vi "Convert_UI_ERD_RT.vi"(0 "New Header?":bool, 2 "ERD Name":string[](array[string]), 5 "All_Bundled_Data_Brass":T1, 7 "Array":T8[](array[typedef]) {"ERD Number" format="%.0x"}, 11 "Error In":errorcluster) -> (6 "All_ERD_Data_Bundled_Brass":T1, 15 "Error Out":errorcluster)   [LabVIEW 2021]
doc: "This VI parses the data from ERDs in correct format, units, etc. It handles all hex to dec conversions, hex to enum, and hex to boolean conversions.\n\nIf Raw Data from ERD is blank string, then it will output values from shift register."
uses:
  Common/LabVIEW GEA2 Toolkit/GEA3/type defs/ERD Read Data Out.ctl
  Controls/All_Bundled_Data_RT.ctl
  Dryer Tool (Commercial 2)/JL Dryer Tool Support/type defs/Version.ctl
  Dryer Tool (Commercial 2)/JL Dryer Tool Support/type defs/ERD_Always_Show_JL.ctl
  Dryer Tool (Commercial 2)/JL Dryer Tool Support/type defs/CSV_File_String_Arrays.ctl
  Dryer Tool (Commercial 2)/JL Dryer Tool Support/type defs/Fault Table Array.ctl
  Dryer Tool (Commercial 2)/JL Dryer Tool Support/type defs/Fault_Table_Info.ctl
  Dryer Tool (Commercial 2)/JL Dryer Tool Support/type defs/BootloaderVersion.ctl
panel:
  out "ERD Number":u16 format="%x"
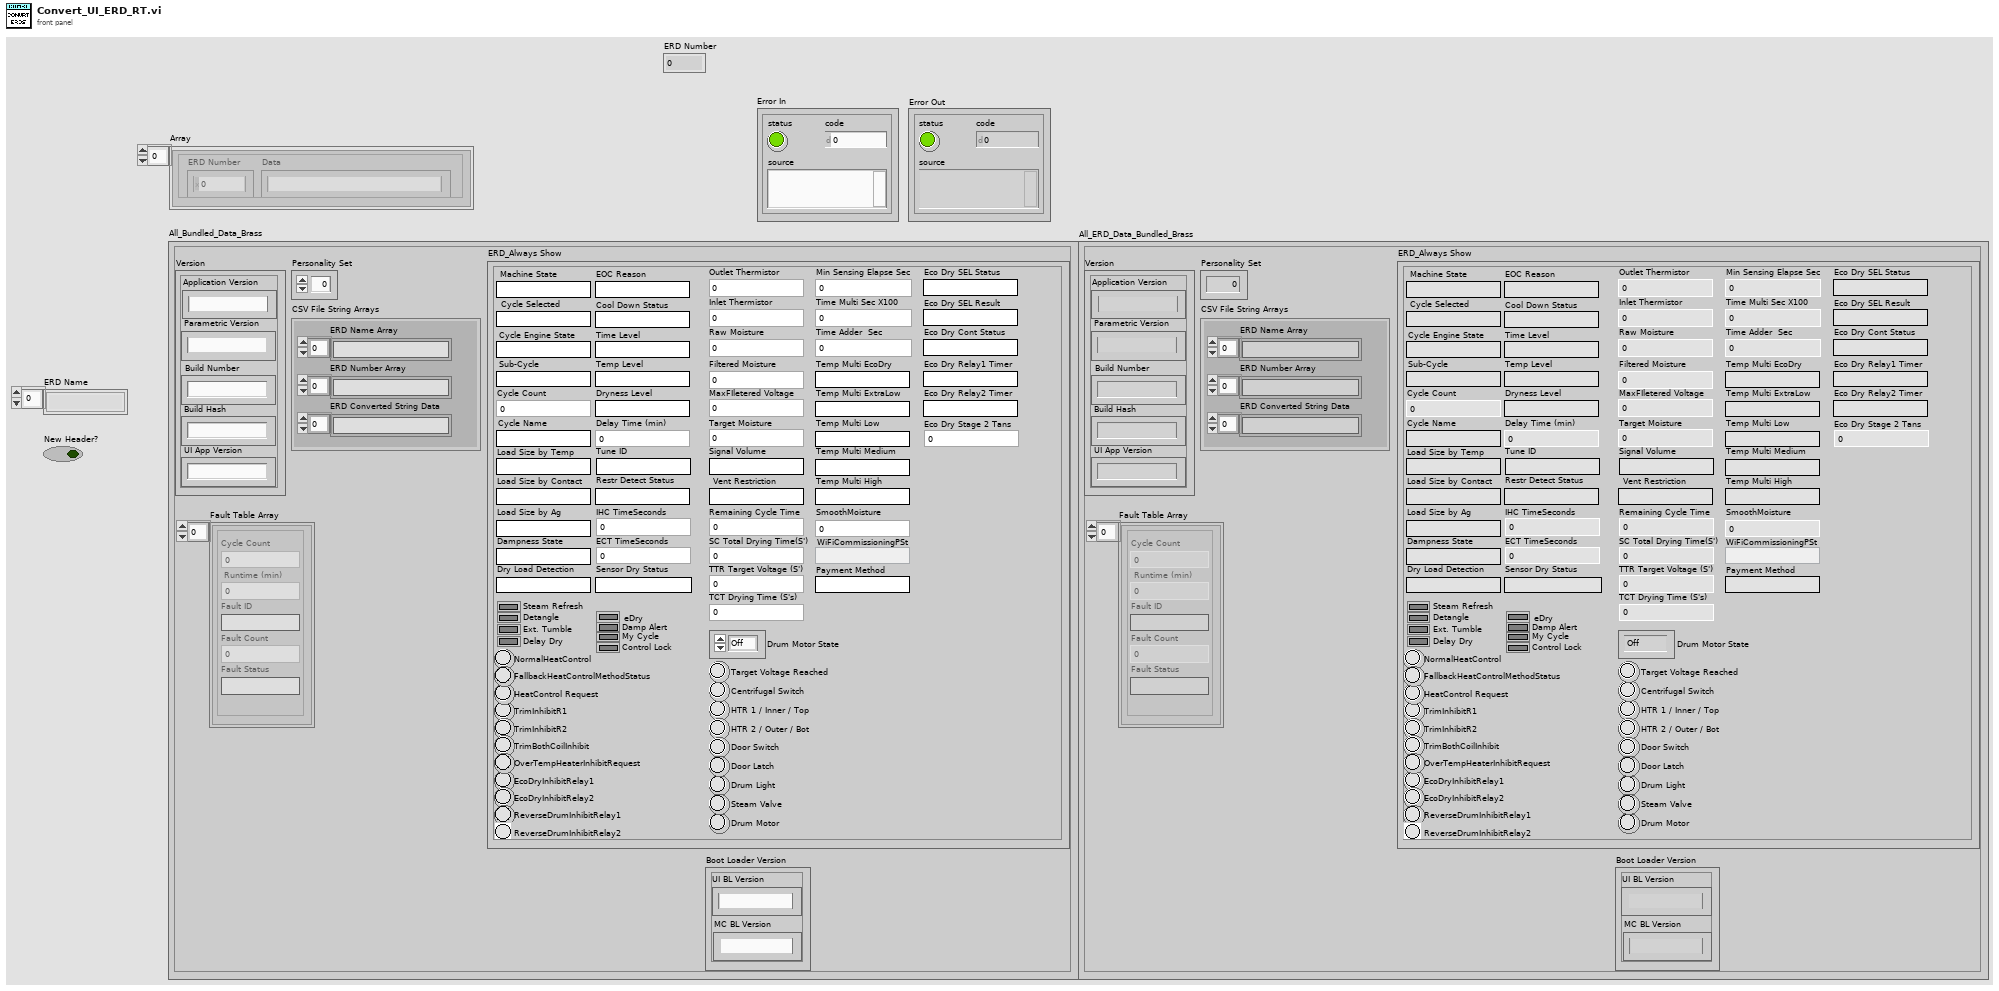
[diagram p1: front panel]
types:
  T1 = typedef "All_Bundled_Data_RT.ctl" = cluster{"Version":T2, "ERD_Always Show":T3, "Personality Set":u8, "CSV File String Arrays":T4, "Fault Table Array ":T5, "Boot Loader Version":T7}
  T2 = typedef "Version.ctl" = cluster{"Build Number":string, "Build Hash ":string, "Application Version":string, "Parametric Version":string, "UI App Version":string}
  T3 = typedef "ERD_Always_Show_JL.ctl" = cluster{"Inlet Thermistor":u16, "Machine State":string, "Filtered Moisture":u16, "Cycle Selected":string, "HTR 1 / Inner / Top":bool, "HTR 2 / Outer / Bot":bool, "Door Switch":bool, "Drum Light":bool, "Cycle Engine State":string, "Centrifugal Switch":bool, "Drum Motor":bool, "Cycle Count":u32, "Ext. Tumble":bool, "eDry":bool, "Temp Level":string, "Dryness Level":string, "Time Level":string, "Delay Time (min)":u16, "Steam Refresh":bool, "Damp Alert":bool, "Sub-Cycle":string, "Outlet Thermistor":u16, "Target Moisture":u16, "Remaining Cycle Time":u32, "Raw Moisture":u16, "Cycle Name":string, "My Cycle":bool, "Delay Dry":bool, "Detangle":bool, "Control Lock":bool, "Steam Valve":bool, "Door Latch":bool, "Signal Volume":string, "Tune ID":string, "Restr Detect Status":string, "Vent Restriction":string, "Load Size by Contact":string, "Load Size by Temp":string, "EOC Reason":string, "Sensor Dry Status":string, "Dampness State":string, "Target Voltage Reached":bool, "TrimInhibitR1":bool, "TrimInhibitR2":bool, "TrimBothCoilInhibit":bool, "NormalHeatControl":bool, "HeatControl Request":bool, "Cool Down Status":string, "EcoDryInhibitRelay1":bool, "EcoDryInhibitRelay2":bool, "ReverseDrumInhibitRelay1":bool, "ReverseDrumInhibitRelay2":bool, "OverTempHeaterInhibitRequest":bool, "FallbackHeatControlMethodStatus":bool, "IHC TimeSeconds":u32, "ECT TimeSeconds ":u32, "SC Total Drying Time(S')":u32, "TTR Target Voltage (S')":u32, "TCT Drying Time (S's)":u32, "Drum Motor State":enum16{"Off", "Cw", "Ccw", "Max"}, "Load Size by Ag":string, "MaxFIletered Voltage":u16, "Dry Load Detection":string, "Min Sensing Elapse Sec":u32, "Time Multi Sec X100":u32, "Time Adder  Sec":u32, "Temp Multi EcoDry":string, "Temp Multi ExtraLow":string, "Temp Multi Low ":string, "Temp Multi Medium":string, "Temp Multi High":string, "SmoothMoisture":u16, "Eco Dry SEL Status":string, "Eco Dry SEL Result":string, "Eco Dry Cont Status":string, "Eco Dry Relay1 Timer":string, "Eco Dry Relay2 Timer ":string, "Eco Dry Stage 2 Tans ":u32, "WiFiCommissioningPSt":string, "Payment Method":string}
  T4 = typedef "CSV_File_String_Arrays.ctl" = cluster{"ERD Number Array":string[], "ERD Name Array":string[], "ERD Converted String Data":string[]}
  T5 = typedef "Fault Table Array.ctl" = T6[]
  T6 = typedef "Fault_Table_Info.ctl" = cluster{"Cycle Count":u32, " Runtime (min) ":u32, "Fault Status":string, "Fault ID":string, "Fault Count":u16}
  T7 = typedef "BootloaderVersion.ctl" = cluster{"UI BL Version":string, "MC BL Version":string}
  T8 = typedef "ERD Read Data Out.ctl" = cluster{"ERD Number":u16, "Data":string}
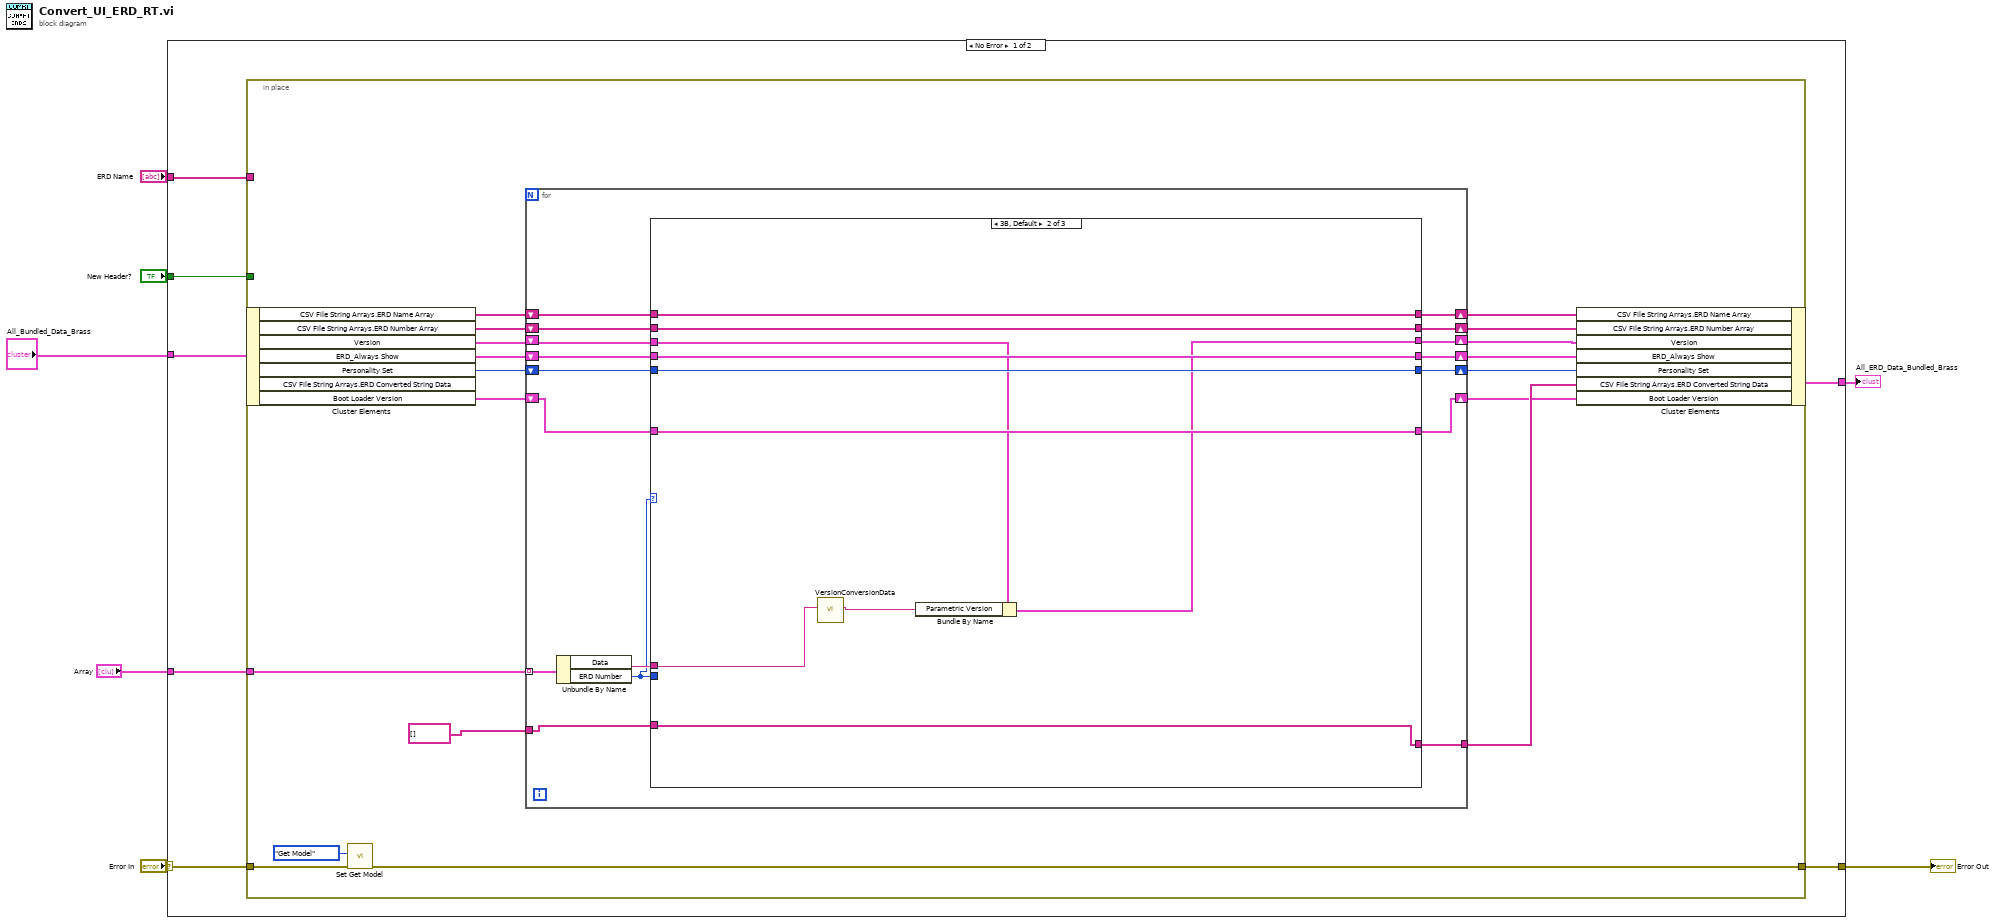
[diagram p0: block diagram]
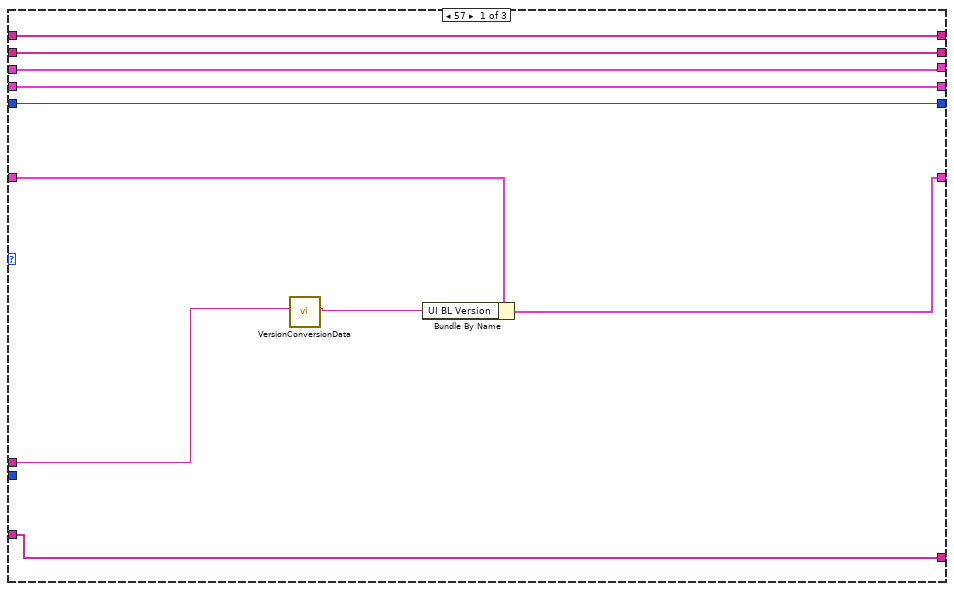
[diagram p2: hidden frame]
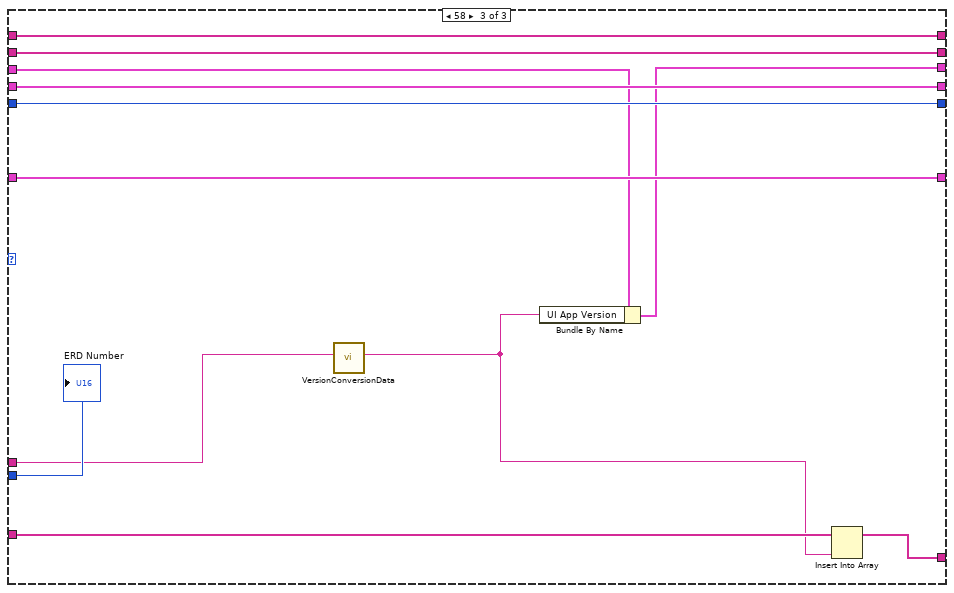
[diagram p3: hidden frame]
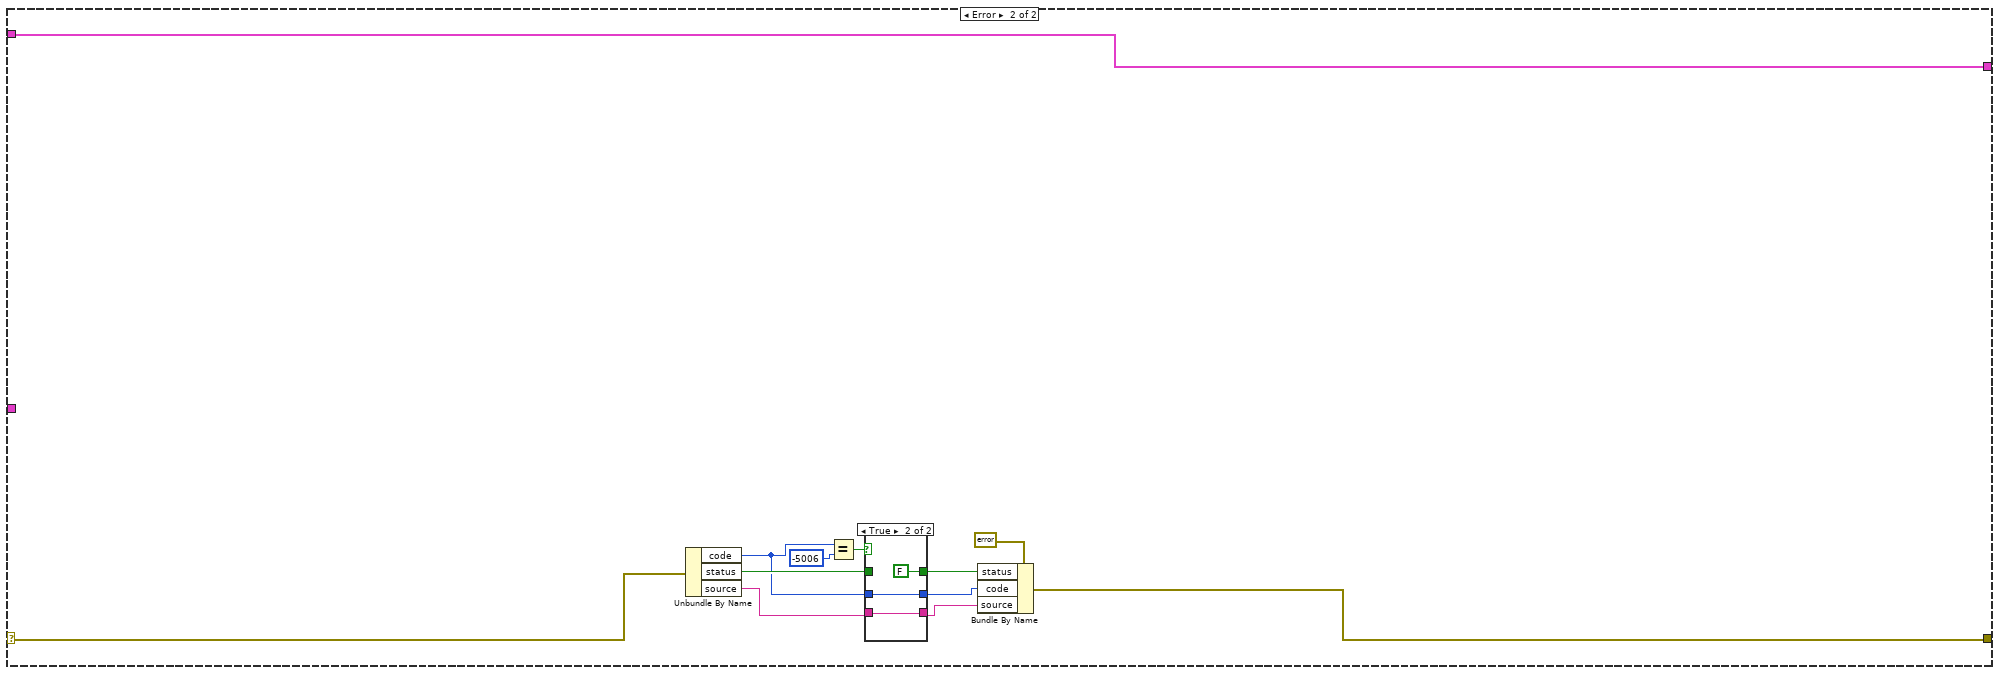
[diagram p4: hidden frame]
diagram:
  n1 = case shown="No Error" "Error In" {
    selector: "Error In" -> [w11 w84]
    tunnel: "Array" -> [w14 _]
    tunnel: [w12 w83] -> w5
    tunnel: "All_Bundled_Data_Brass" -> [w13 w82]
    tunnel: [w10 w82] -> w1
    tunnel: "New Header?" -> [w9 _]
    tunnel: "ERD Name" -> [w8 _]
    frame No Error {
      n2 = in-place {
        in-place-border: w14 -> [w27]
        in-place-border: [w29] -> w12
        in-place-border: w11 -> [w30]
        in-place-border: w9 -> [_]
        in-place-border: w8 -> [_]
        n3 = in-place-cluster #1(w13) -> ("CSV File String Arrays.ERD Name Array"=w18:string[], "CSV File String Arrays.ERD Number Array"=w17:string[], "Version"=w21:T2, "ERD_Always Show"=w22:T3, "Personality Set"=w24:u8, "Boot Loader Version"=w25:T7)  [unwired: 1 out]
        n4 = call "Set Get Model.vi"("Error In"=w30, "Action"=enum16{"Set Model", "Get Model"}."Get Model") -> ("Error Out"=w29:errorcluster)  [unwired: 8 in, 1 out]
        n5 = for {
          tunnel: string[] [] ("ERD String Data") -> [w46]
          tunnel: [w49] -> w31
          tunnel: w27 -> [w47] mode=indexing
          shift-right: [w43] -> w26
          shift-left: w25 -> [w44]
          shift-right: [w36] -> w19
          shift-left: w18 -> [w35]
          shift-right: [w33] -> w16
          shift-left: w17 -> [w34]
          shift-right: [w37] -> w20
          shift-left: w21 -> [w38]
          shift-right: [w39] -> w15
          shift-left: w22 -> [w40]
          shift-right: [w41] -> w23
          shift-left: w24 -> [w42]
          n6 = Unbundle By Name(w47) -> ("Data"=w48:string, "ERD Number"=w45:u16)
          n7 = case shown="3B, Default" w45 {
            tunnel: [w59 w64 w81] -> w49
            tunnel: w48 -> [w51 w62 w71]
            tunnel: w45 -> [_ _ w80]
            tunnel: w46 -> [w59 w64 w79]
            tunnel: w44 -> [w58 w65 w74]
            tunnel: [w57 w65 w74] -> w43
            tunnel: w42 -> [w56 w66 w75]
            tunnel: [w56 w66 w75] -> w41
            tunnel: w40 -> [w55 w67 w76]
            tunnel: [w55 w67 w76] -> w39
            tunnel: w38 -> [w54 w61 w73]
            tunnel: [w54 w60 w72] -> w37
            tunnel: [w53 w69 w78] -> w36
            tunnel: w35 -> [w53 w69 w78]
            tunnel: w34 -> [w52 w68 w77]
            tunnel: [w52 w68 w77] -> w33
            frame 57 {
              n8 = call "VersionConversionData.vi"("Version In"=w51) -> ("Version Out"=w50:string)  [unwired: 9 in, 1 out]
              n9 = Bundle By Name(cluster=w58, "UI BL Version"=w50) -> (w57:T7)
            }
            frame 59, Default {
              n10 = call "VersionConversionData.vi"("Version In"=w62) -> ("Version Out"=w63:string)  [unwired: 9 in, 1 out]
              n11 = Bundle By Name(cluster=w61, "Parametric Version"=w63) -> (w60:T2)
            }
            frame 58 {
              n12 = call "VersionConversionData.vi"("Version In"=w71) -> ("Version Out"=w70:string)  [unwired: 9 in, 1 out]
              n13 = Bundle By Name(cluster=w73, "UI App Version"=w70) -> (w72:T2)
              n14 = Insert Into Array(array=w79, new element=w70) -> (w81:string[])  [unwired: 1 in]
              "ERD Number" <- w80
            }
          }
        }
        n15 = in-place-cluster #1("CSV File String Arrays.ERD Name Array"=w19, "CSV File String Arrays.ERD Number Array"=w16, "Version"=w20, "ERD_Always Show"=w15, "Personality Set"=w23, "CSV File String Arrays.ERD Converted String Data"=w31, "Boot Loader Version"=w26) -> (w10:T1)
      }
    }
    frame Error {
      n16 = Unbundle By Name(w84) -> ("code"=w88:i32, "status"=w89:bool, "source"=w86:string)
      n17 = Equal?(x=w88, y=-5006) -> (x = y?=w92:bool)
      n18 = case shown="True" w92 {
        tunnel: [w96 FALSE] -> w90
        tunnel: w89 -> [w96 _]
        tunnel: w88 -> [w95 w98]
        tunnel: [w95 w98] -> w87
        tunnel: [w94 w97] -> w85
        tunnel: w86 -> [w94 w97]
        frame False {
        }
        frame True {
        }
      }
      n19 = Bundle By Name(cluster=errorcluster {"status"=FALSE, "code"=0, "source"=""} ("error constant"), "status"=w90, "code"=w87, "source"=w85) -> (w83:errorcluster)
    }
  }
  "Error Out" <- w5
  "All_ERD_Data_Bundled_Brass" <- w1
